vi "Init.vi"(8 "error in (no error)":errorcluster, 11 "Domain_Evolut_1D":refnum<class "NI_Domain_Evolut_1D.lvclass">) -> (0 "error out":errorcluster, 3 "initialized Domain_Evolut_1D":refnum<class "NI_Domain_Evolut_1D.lvclass">)   [LabVIEW 2017, in "NI_PDE.lvlib" / "NI_Domain_Evolut_1D.lvclass"]
uses:
  <vilib>/gmath/pde.llb/DomainClass/Domain_Evolut_1D/NI_Domain_Evolut_1D.lvclass
  <vilib>/gmath/pde.llb/DomainClass/Class Type.ctl
  <vilib>/gmath/pde.llb/DomainClass/Domain_Evolut_1D/NI_Domain_Evolut_1D.lvclass/NI_Domain_Evolut_1D.ctl
  <vilib>/gmath/pde.llb/DomainClass/Domain_Evolut/NI_Domain_Evolut.lvclass
  <vilib>/gmath/pde.llb/DomainClass/NI_Domain.lvclass
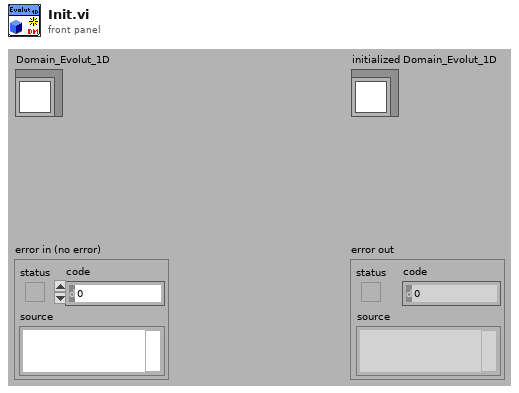
[diagram p1: front panel]
types:
  T1 = cluster{"start x":dbl, "end x":dbl, "# of x-points":i32}
  T2 = typedef "NI_PDE.lvlib/NI_Domain.lvclass/Class Type.ctl" = i32
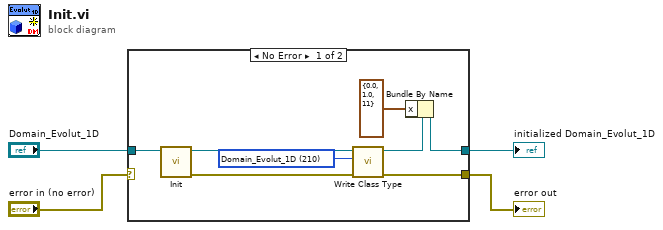
[diagram p0: block diagram]
diagram:
  n1 = case shown="No Error" "error in (no error)" {
    selector: "error in (no error)" -> [_ w14]
    tunnel: [w10 w13] -> w4
    tunnel: [w9 w14] -> w3
    tunnel: "Domain_Evolut_1D" -> [w5 w13]
    frame No Error {
      w12 = T2 210 items=["Domain"=0, "Domain_Steady"=100, "Domain_Steady_2D_Rect"=121, "Domain_Steady_2D_Polygon"=122, "Domain_Evolut"=200, "Domain_Evolut_1D"=210, "Domain_Evolut_2D_Rect"=221] ("domain class type")
      n2 = call-parent "Init.vi"("Domain_Evolut"=w5) -> ("error out"=w7:errorcluster, "initialized Domain_Evolut"=w6:refnum<class "NI_Domain_Evolut_1D.lvclass">)  [unwired: 1 in, 8 out]
      n3 = call-dynamic "Write Class Type.vi"("error in (no error)"=w7, "domain class type"=w12, "Domain.lvclass in"=w6) -> ("error out"=w9:errorcluster, "Domain.lvclass out"=w11:refnum<class "NI_Domain_Evolut_1D.lvclass">)  [unwired: 7 out]
      n4 = Bundle By Name(cluster=w11, "x"=T1 {"start x"=0.0, "end x"=1.0, "# of x-points"=11}) -> (w10:refnum<class "NI_Domain_Evolut_1D.lvclass">)
    }
    frame Error {
    }
  }
  "initialized Domain_Evolut_1D" <- w4
  "error out" <- w3
